vi "LVClass_Pupil ctor from txt file.vi"(0 "Pupil (const)":refnum<class "Pupil.lvclass">, 5 "file path txt":path, 7 "Dimensions_µm":T1, 11 "error in (no error)":errorcluster) -> (4 "Pupil (new)":refnum<class "Pupil.lvclass">, 15 "error out":errorcluster)   [LabVIEW 2020, in "Pupil.lvclass"]
doc: "Circular Pupil constructor from dimensions, steps and circle shape.\n\n--------------------------------------------------------------------------------\n\n<B>PupilIn </B> : Constant Pointer to Pupil object.\n<B>PupilOut </B> : Constant Pointer to Pupil object.\n<B>step </B> : Step x and y between the subpupils (um).\n<B>dimensions </B> : Pupil array dimensions (width, height).\n<B>center </B> : Center of the circle shape (um).\n<B>radius </B> : Radius of the circle shape (um).\n<B>ErrorIn </B> : Error\n<B>ErrorOut </B> : Error\n\n--------------------------------------------------------------------------------"
uses:
  Pupil.lvclass
  General dimensions definition.ctl
  Point2D.ctl
  Point2Df.ctl
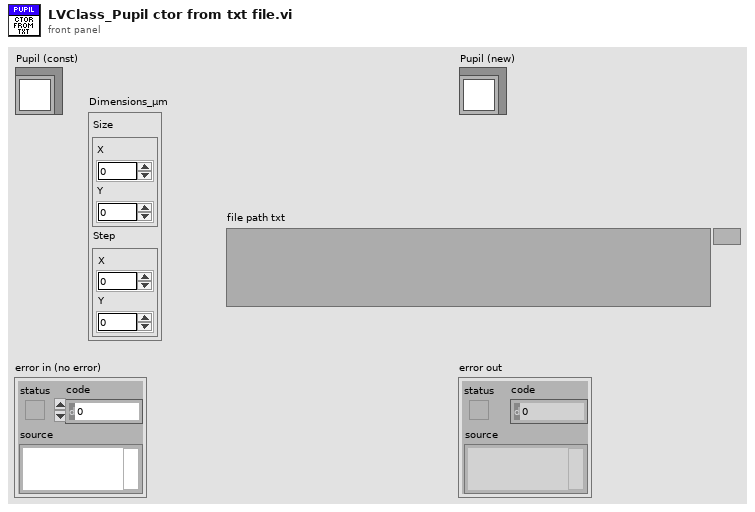
[diagram p1: front panel]
types:
  T1 = typedef "General dimensions definition.ctl" = cluster{"Size":T2, "Step":T3}
  T2 = typedef "Point2D.ctl" = cluster{"X":u32, "Y":u32}
  T3 = typedef "Point2Df.ctl" = cluster{"X":sgl, "Y":sgl}
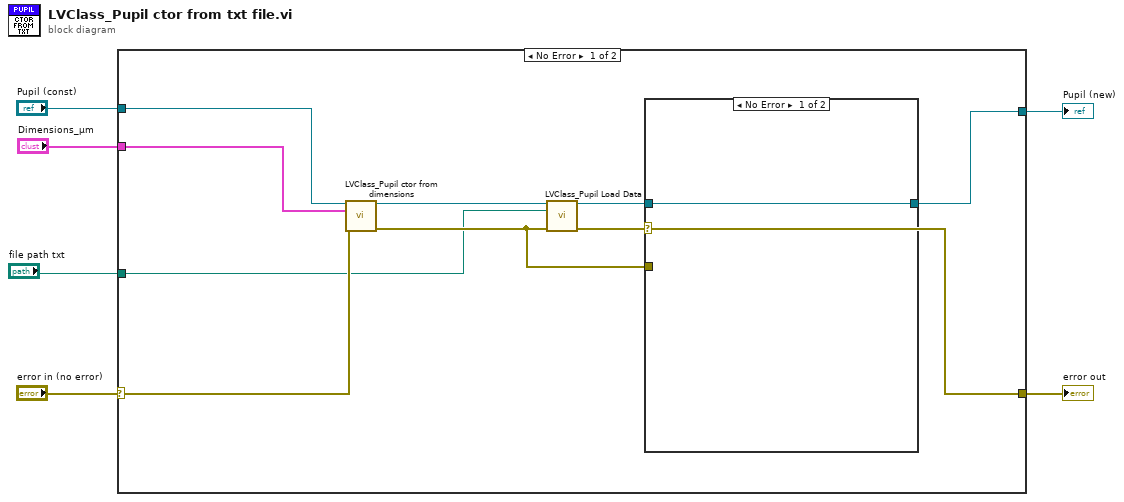
[diagram p0: block diagram]
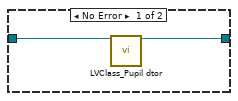
[diagram p3: hidden frame]
diagram:
  n1 = case shown="No Error" "error in (no error)" {
    selector: "error in (no error)" -> [w13 w24]
    tunnel: [w9 w24] -> w5
    tunnel: [w8 w23] -> w3
    tunnel: "Pupil (const)" -> [w15 w23]
    tunnel: "Dimensions_µm" -> [w14 _]
    tunnel: "file path txt" -> [w7 _]
    frame No Error {
      n2 = call "LVClass_Pupil ctor from dimensions.vi"("Pupil (const)"=w15, "Dimensions_um"=w14, "error in (no error)"=w13) -> ("Pupil (new)"=w12:refnum<class "Pupil.lvclass">, "error out"=w11:errorcluster)  [unwired: 11 in]
      n3 = call "LVClass_Pupil Load Data.vi"("Pupil in"=w12, "file path txt"=w7, "error in (no error)"=w11) -> ("Pupil out"=w10:refnum<class "Pupil.lvclass">, "error out"=w9:errorcluster)  [unwired: 11 in]
      n4 = case shown="No Error" w9 {
        tunnel: w11 -> [_ w19]
        tunnel: w10 -> [w16 w18]
        tunnel: [w16 w17] -> w8
        frame No Error {
        }
        frame Error {
          n5 = case shown="Error" w19 {
            tunnel: w18 -> [w21 w22]
            tunnel: [w20 w22] -> w17
            frame No Error {
              n6 = call "LVClass_Pupil dtor.vi"("Pupil in"=w21) -> ("Pupil out"=w20:refnum<class "Pupil.lvclass">)  [unwired: 13 in, 1 out]
            }
            frame Error {
            }
          }
        }
      }
    }
    frame Error {
    }
  }
  "error out" <- w5
  "Pupil (new)" <- w3
